vi "ZLIB Common Path to Specific Path__ogtk.vi"(10 "common path":string) -> (2 "specific path":path)   [LabVIEW 2014]
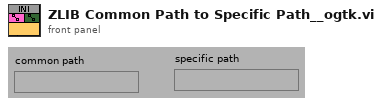
[diagram p1: front panel]
types:
  T1 = enum32{"invalid OS target", "Mac OS", "Windows 3.1", "Windows 95/NT", "Solaris 1", "Solaris 2", "HP-UX", "PowerMAX", "Linux", "Irix", "Rhapsody", "BeOS", "AIX", "OSF1", "VxWorks", "PharLap", "Carbon", "RTX", "Windows x64", "Linux x64", "Mac OS X x64"}
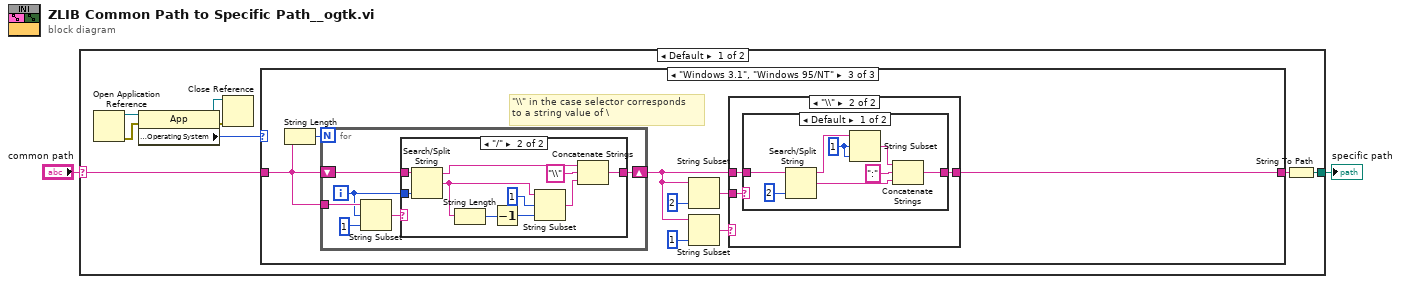
[diagram p0: block diagram]
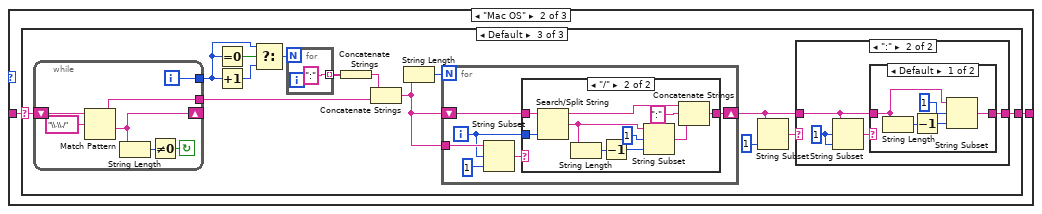
[diagram p3: hidden frame]
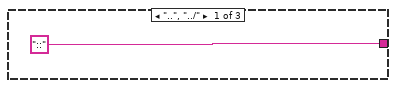
[diagram p4: hidden frame]
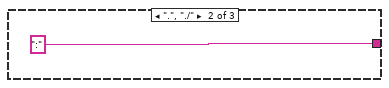
[diagram p5: hidden frame]
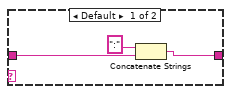
[diagram p7: hidden frame]
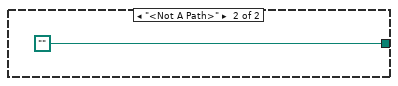
[diagram p12: hidden frame]
diagram:
  n1 = case shown="Default" "common path" {
    selector: "common path" -> [w10 _]
    tunnel: [w9 path "" ("Not A Path Constant")] -> w1
    frame Default {
      n2 = Open Application Reference() -> (0:w3:errorcluster, 3:w4:refnum<vi>)  [unwired: 4 in]
      n3 = property class="App"(reference=w4, error in=w3) -> (reference out=w5:refnum<vi>, error out=w6:errorcluster, "Application:Target:Operating System"=w7:T1)
      n4 = Close Reference(reference=w5, error in (no error)=w6) -> ()  [unwired: 1 out]
      n5 = case shown="\"Windows 3.1\", \"Windows 95/NT\"" w7 {
        tunnel: w10 -> [w11 w13 w75]
        tunnel: [w11 w12 w73] -> w8
        frame "invalid OS target", Default {
        }
        frame "Mac OS" {
          n6 = case shown="Default" w13 {
            selector: w13 -> [_ _ w19]
            tunnel: ["::" ":" w18] -> w12
            frame "..", "../" {
            }
            frame ".", "./" {
            }
            frame Default {
              n7 = while {
                shift-right: [w31] -> _
                shift-left: w19 -> [w35]
                tunnel: [w32] -> w23
                tunnel: [w30] -> w27
                i -> [w30]
                stop <- w33 continue-if-true
                n8 = Match Pattern(string=w35, regular expression="\\.\\./") -> (before substring=w32:string, after substring=w31:string)  [unwired: 3 out]
                n9 = String Length(string=w31) -> (length=w34:i32)
                n10 = Not Equal To 0?(x=w34) -> (x != 0?=w33:bool)
              }
              n11 = Equal To 0?(x=w27) -> (x = 0?=w28:bool)
              n12 = Increment(x=w27) -> (x+1=w26:i32)
              n13 = Select(t=w27, s=w28, f=w26) -> (s? t:f=w25:i32)
              n14 = for {
                N: w25 -> [_]
                tunnel: [":"] -> w24 mode=indexing
              }
              n15 = Concatenate Strings(w24) -> (w17:string)
              n16 = Concatenate Strings(w17, w23) -> (w21:string)
              n17 = String Length(string=w21) -> (length=w22:i32)
              n18 = for {
                N: w22 -> [_]
                tunnel: w21 -> [w40]
                shift-right: [w41] -> w16
                shift-left: w21 -> [w42]
                i -> [w39]
                n19 = String Subset(string=w40, offset (0)=w39, length (rest)=1 ("length")) -> (substring=w37:string)
                n20 = case shown="\"/\"" w37 {
                  tunnel: w42 -> [w43 w53]
                  tunnel: w39 -> [_ w46]
                  tunnel: [w43 w51] -> w41
                  frame Default {
                  }
                  frame "/" {
                    n21 = Search/Split String(string=w53, offset (0)=w46) -> (substring before match=w52:string, match + rest of string=w45:string)  [unwired: 2 out]
                    n22 = String Length(string=w45) -> (length=w49:i32)
                    n23 = Decrement(x=w49) -> (x-1=w48:i32)
                    n24 = String Subset(string=w45, offset (0)=1, length (rest)=w48) -> (substring=w44:string)
                    n25 = Concatenate Strings(w52, ":" ("x"), w44) -> (w51:string)
                  }
                }
              }
              n26 = String Subset(string=w16, length (rest)=1 ("length")) -> (substring=w20:string)  [unwired: 1 out]
              n27 = case shown="\":\"" w20 {
                tunnel: w16 -> [w57 w60]
                tunnel: [w56 w61] -> w18
                frame Default {
                  n28 = Concatenate Strings(":", w57) -> (w56:string)
                }
                frame ":" {
                  w59 = 1 ("length")
                  n29 = String Subset(string=w60, offset (0)=w59, length (rest)=w59) -> (substring=w58:string)
                  n30 = case shown="Default" w58 {
                    tunnel: w60 -> [w62 w67]
                    tunnel: [w63 w67] -> w61
                    frame Default {
                      n31 = String Length(string=w62) -> (length=w65:i32)
                      n32 = Decrement(x=w65) -> (x-1=w64:i32)
                      n33 = String Subset(string=w62, offset (0)=1, length (rest)=w64) -> (substring=w63:string)
                    }
                    frame ":" {
                    }
                  }
                }
              }
            }
          }
        }
        frame "Windows 3.1", "Windows 95/NT" {
          # "\"\\\\\" in the case selector corresponds\nto a string value of \\"
          n34 = String Length(string=w75) -> (length=w71:i32)
          n35 = for {
            N: w71 -> [_]
            tunnel: w75 -> [w79]
            shift-right: [w80] -> w70
            shift-left: w75 -> [w81]
            i -> [w78]
            n36 = String Subset(string=w79, offset (0)=w78, length (rest)=1 ("length")) -> (substring=w76:string)
            n37 = case shown="\"/\"" w76 {
              tunnel: w81 -> [w82 w92]
              tunnel: w78 -> [_ w84]
              tunnel: [w82 w90] -> w80
              frame Default {
              }
              frame "/" {
                n38 = Search/Split String(string=w92, offset (0)=w84) -> (substring before match=w91:string, match + rest of string=w88:string)  [unwired: 2 out]
                n39 = String Length(string=w88) -> (length=w87:i32)
                n40 = Decrement(x=w87) -> (x-1=w86:i32)
                n41 = String Subset(string=w88, offset (0)=1, length (rest)=w86) -> (substring=w83:string)
                n42 = Concatenate Strings(w91, "\\" ("x"), w83) -> (w90:string)
              }
            }
          }
          n43 = String Subset(string=w70, length (rest)=2 ("length")) -> (substring=w68:string)  [unwired: 1 out]
          n44 = String Subset(string=w70, length (rest)=1 ("length")) -> (substring=w69:string)  [unwired: 1 out]
          n45 = case shown="\"\\\\\"" w69 {
            tunnel: w70 -> [w93 w96]
            tunnel: [w93 w95] -> w73
            tunnel: w68 -> [_ w94]
            frame Default {
            }
            frame "\\" {
              n46 = case shown="Default" w94 {
                tunnel: w96 -> [w104 w105]
                tunnel: [w98 w105] -> w95
                frame Default {
                  w97 = 1 ("offset (0)")
                  n47 = Search/Split String(string=w104, offset (0)=2) -> (substring before match=w102:string, match + rest of string=w99:string)  [unwired: 2 out]
                  n48 = String Subset(string=w102, offset (0)=w97, length (rest)=w97) -> (substring=w101:string)
                  n49 = Concatenate Strings(w101, ":", w99) -> (w98:string)
                }
                frame "\\\\" {
                  # "\"\\\\\\\\\" in the case selector corresponds\nto a string value of \\\\"
                }
              }
            }
          }
        }
      }
      n50 = String To Path(string=w8) -> (path=w9:path)
    }
    frame "<Not A Path>" {
    }
  }
  "specific path" <- w1
